vi "Object Tracking.vi"() -> ()   [LabVIEW 2015]
panel:
  out "Objects (real-world) (Object Tracking 1)":T1(array[cluster])
  out "Objects (pixel) (Object Tracking 1)":T1(array[cluster])
  out "Image Out 2":T2(plugin-control)
  in  "stop":bool
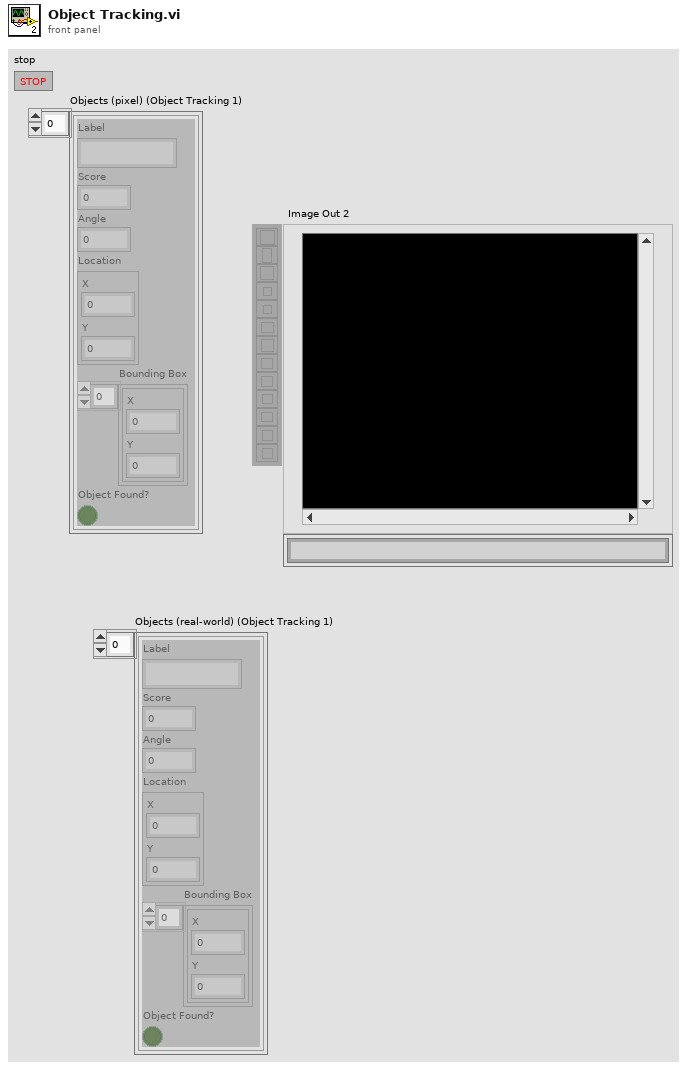
[diagram p1: front panel]
types:
  T1 = cluster{"Label":string, "Score":i32, "Angle":dbl, "Location":cluster{"X":dbl, "Y":dbl}, "Bounding Box":cluster{"X":dbl, "Y":dbl}[], "Object Found?":bool}[]
  T2 = typedef "IMAQ Image.ctl" = refnum<image>
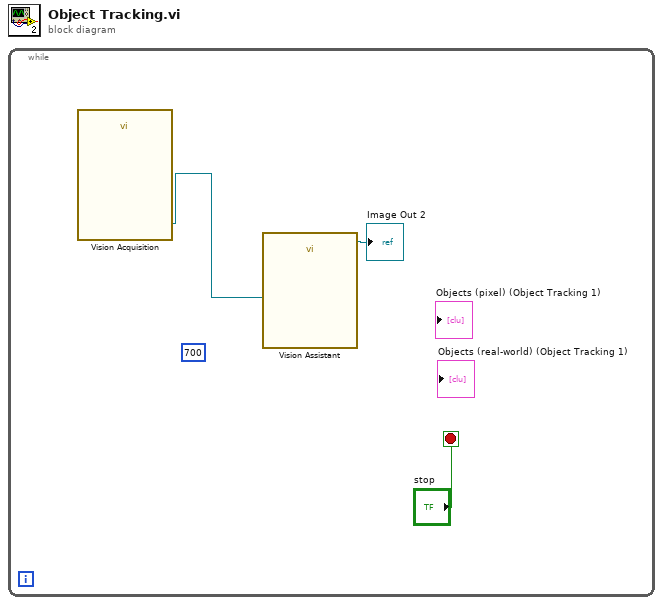
[diagram p0: block diagram]
diagram:
  n1 = while {
    stop <- "stop" stop-if-true
    (unwired) 700
    n2 = call "Vision Acquisition"() -> ("Image Out"=w1:T2)  [unwired: 25 in, 2 out]
    n3 = call "Vision Assistant"("Image In"=w1) -> ("Image Out"=→"Image Out 2":T2)  [unwired: 25 in, 1 out]
  }
